vi "Error Case Strings.vi"() -> (1 "Error":string, 3 "No Error":string)   [LabVIEW 2017]
uses:
  _Shared/CSM Shared.lvlib
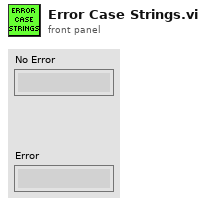
[diagram p1: front panel]
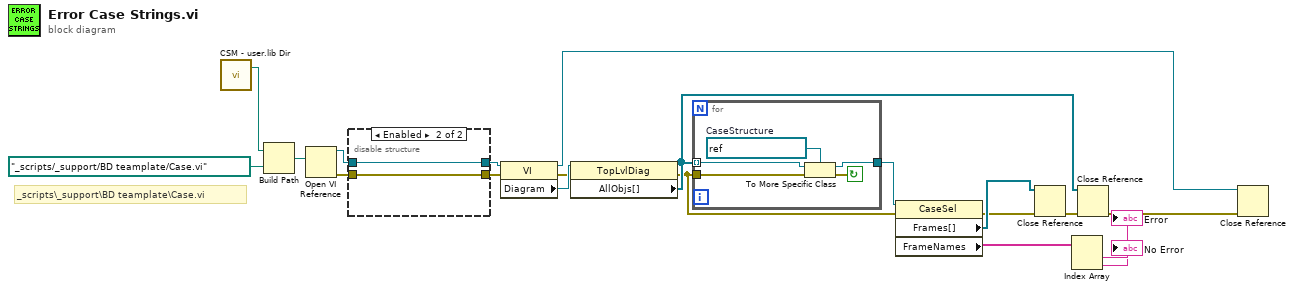
[diagram p0: block diagram]
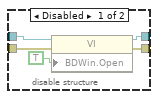
[diagram p2: hidden frame]
diagram:
  # "_scripts\\_support\\BD teamplate\\Case.vi"
  n1 = call "CSM - user.lib Dir.vi"() -> ("csm_user.lib_dir"=w8:path)  [unwired: 2 in, 1 out]
  n2 = Build Path ("创建路径")(base path=w8, name or relative path=path "_scripts/_support/BD teamplate/Case.vi") -> (appended path=w9:path)
  n3 = Open VI Reference ("打开VI引用")(vi path=w9) -> (vi reference=w7:refnum<vi>, error out=w6:errorcluster)  [unwired: 5 in]
  n4 = disable-structure "程序框图禁用结构" shown="Enabled" {
    disable-tunnel: w7 -> [w25 w27]
    disable-tunnel: w6 -> [w24 w26]
    disable-tunnel: [w23 w27] -> w19
    disable-tunnel: [w22 w26] -> w18
    frame Disabled {
      n5 = property class="VI"(reference=w25, error in=w24, "BDWin.Open"=TRUE ("Block Diagram Window:Open")) -> (reference out=w23:refnum<vi>, error out=w22:errorcluster)
    }
    frame Enabled {
    }
  }
  n6 = property on="属性节点" class="VI"(reference=w19, error in=w18) -> (reference out=w14:refnum<vi>, error out=w16:errorcluster, "Diagram"=w17:refnum<vi>)
  n7 = property on="属性节点" class="TopLvlDiag"(reference=w17, error in=w16) -> (error out=w12:errorcluster, "AllObjs[]"=w13:refnum<vi>[])  [unwired: 1 out]
  n8 = for "For循环" {
    tunnel: w13 -> [w32] mode=indexing
    tunnel: [w28] -> w15
    tunnel: w12 -> [w30]
    stop <- w29 continue-if-true
    w31 = refnum<vi> refnum  # CaseStructure
    n9 = To More Specific Class(target class=w31, reference=w32, error in=w30) -> (specific class reference=w28:refnum<vi>, error out=w29:errorcluster)
  }
  n10 = property on="属性节点" class="CaseSel"(reference=w15, error in=w12) -> (error out=w5:errorcluster, "Frames[]"=w11:refnum<vi>[], "FrameNames"=w3:string[])  [unwired: 1 out]
  n11 = Close Reference ("关闭引用")(reference=w11, error in (no error)=w5) -> (error out=w10:errorcluster)
  n12 = Index Array ("索引数组")(array=w3) -> (element #1=→"No Error":string, element #2=→"Error":string)  [unwired: 2 in]
  n13 = Close Reference ("关闭引用")(reference=w13, error in (no error)=w10) -> (error out=w4:errorcluster)
  n14 = Close Reference ("关闭引用")(reference=w14, error in (no error)=w4) -> ()  [unwired: 1 out]
